vi "Multiple Sessions with a Raspberry Pi.vi"() -> ()   [LabVIEW 2018]
doc: "Creates multiple, parallel sessions with a Raspberry Pi."
uses:
  Toolkit/Channel/Channel.lvclass/Channel.ctl
  Toolkit/Session/Session.lvclass/Session.ctl
  Toolkit/SSH/SSH.lvclass/SSH.ctl
  Toolkit/Session/Utility/Read Shared Library.vi
  Toolkit/SSH/Utility/Read Shared Library.vi
  Toolkit/Session/Support/Create from SSH.vi
  Toolkit/Session/Support/Password Authentication.vi
  Toolkit/Channel/Support/Create from Session.vi
  Toolkit/Support/Check Status.vi
  Toolkit/Channel/Support/Destroy to Session.vi
  Toolkit/Session/Support/Destroy to SSH.vi
  Toolkit/SSH/SSH.lvclass
  Toolkit/Session/Session.lvclass
  Toolkit/Channel/Channel.lvclass
panel:
  out "Login Message Size 2":i32 caption="Login Size"
  out "Login Message 2":string
  out "Login Message Size 1":i32 caption="Login Size"
  in  "Max Login Message Size":u64=1024 caption="Max Login Size"
  out "Response 2 Size":i32 caption="Response Size"
  in  "Command 2 Max Response Size":u64=1024 caption="Max Response Size"
  out "Response 1 Size":i32 caption="Response Size"
  in  "Command 1 Max Response Size":u64=1024 caption="Max Response Size"
  in  "Timeout":i32=1000 caption="Timeout (ms)"
  out "Login Message 1":string
  out "Response 2":string
  in  "Command 2":string="echo \"Hello World from the second command!\""
  out "Response 1":string
  in  "Command 1":string="echo \"Hello World from the first command!\""
  in  "Raspberry Pi Address":string="raspberrypi.local"
  in  "Password":string
  in  "Username":string="pi"
  # "Overview: Demonstrates creating multiple, parallel sessions with a Raspberry Pi\nInstructions:\n1. Change the Raspberry Pi Address from the mDNS default to another mDNS or the IP address of the Raspberry Pi if needed.\n2. Change the username from the default Raspberry Pi user if needed.\n3. Enter the password for the Raspberry Pi user.\n4. Run this VI.\n5. Observe the login message from the Raspberry Pi.\n6. Observe \"Hello World from the first command!\" and \"Hello World from the second command!\" for Response 1 and 2, respectively.\n7. Change Command 1 and Command 2.\n8. Rerun this VI.\n9. Observe the responses for Command 1 and Command 2, respectively."
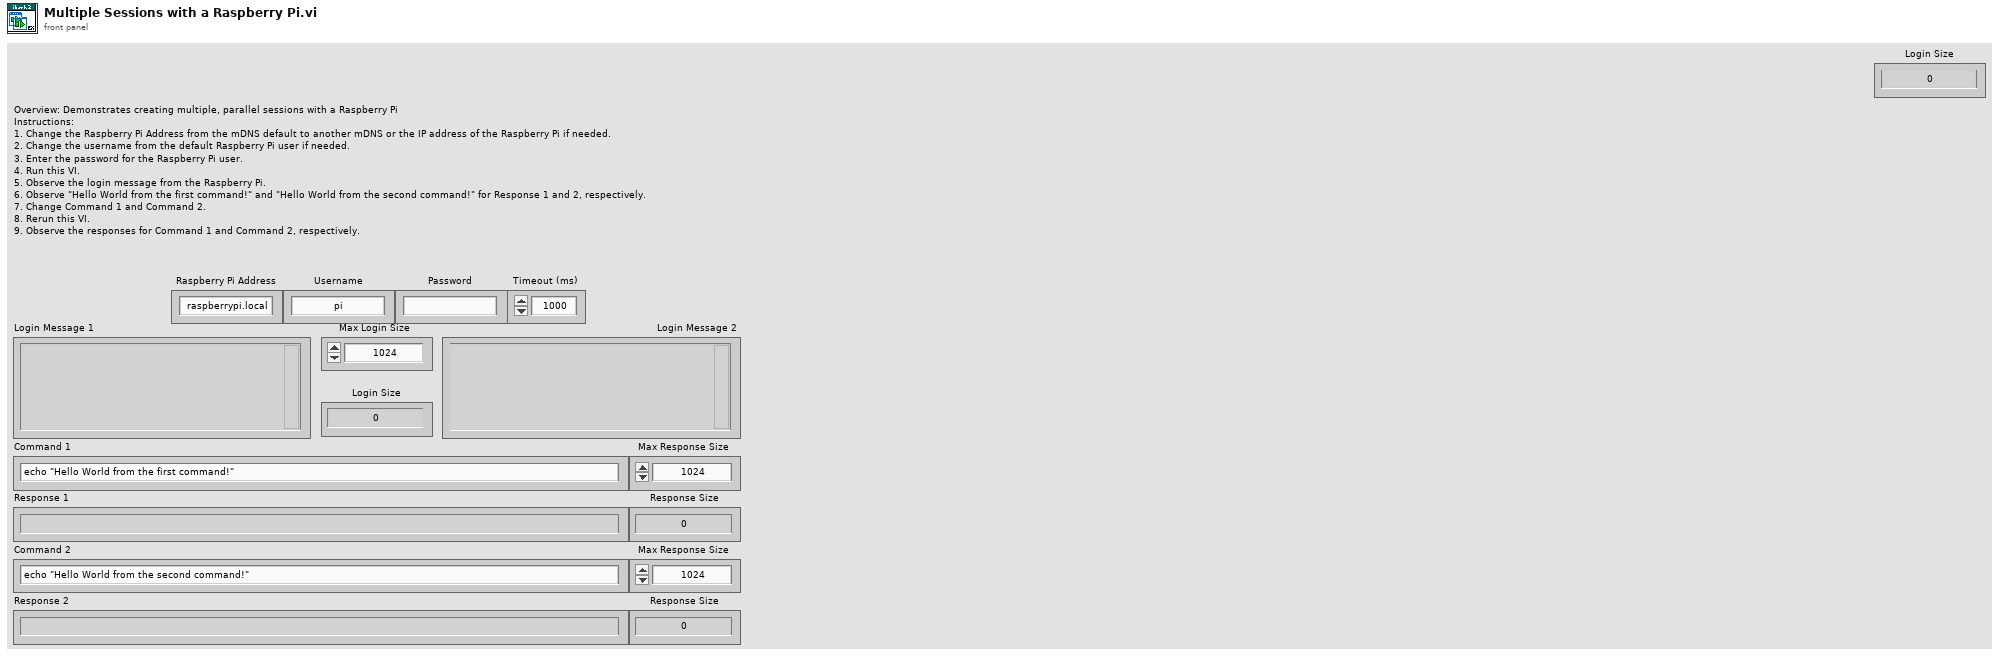
[diagram p1: front panel]
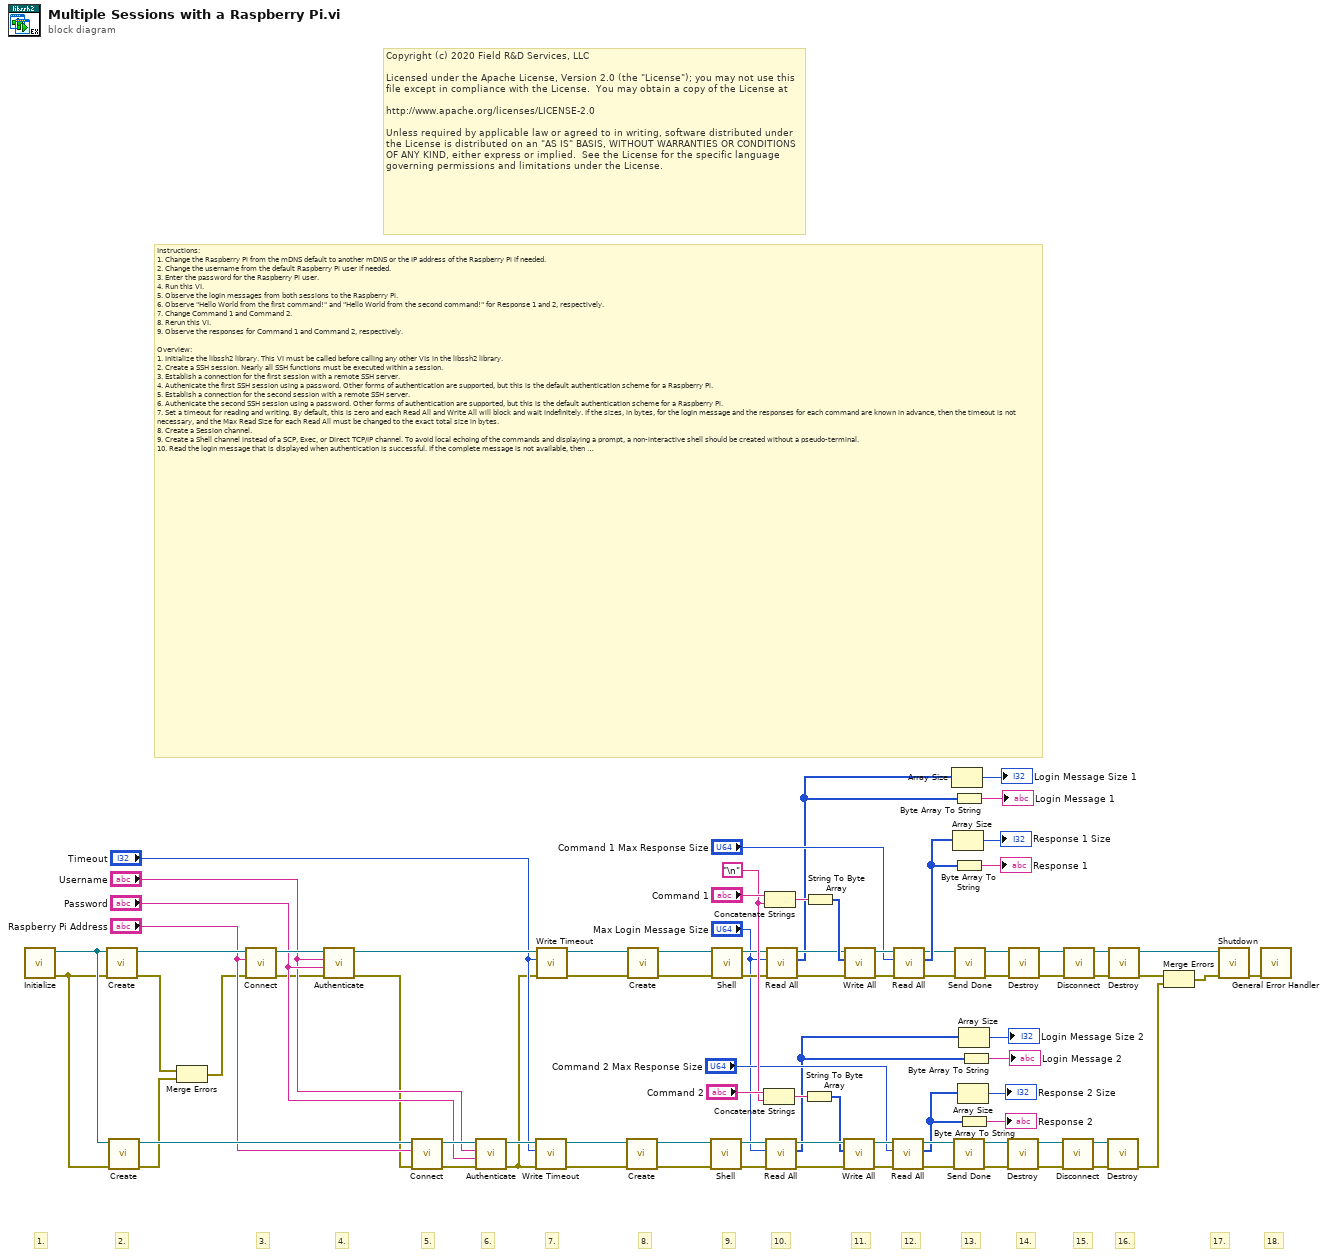
[diagram p0: block diagram]
diagram:
  w62 = "\n"
  # "18."
  # "17."
  # "16."
  # "Copyright (c) 2020 Field R&D Services, LLC\n\nLicensed under the Apache License, Version 2.0 (the \"License\"); you may not use this file except in compliance with the License.  You may obtain a copy of the License at\n\nhttp://www.apache.org/licenses/LICENSE-2.0\n\nUnless required by applicable law or agreed to in writing, software distributed under the License is distributed on an \"AS IS\" BASIS, WITHOUT WARRANTIES OR CONDITIONS OF ANY KIND, either express or implied.  See the License for the specific language governing permissions and limitations under the License."
  # "15."
  # "14."
  # "13."
  # "12."
  # "11."
  # "10."
  # "9."
  # "8."
  # "7."
  # "6."
  # "5."
  # "4."
  # "3."
  # "2."
  # "1."
  # "Instructions:\n1. Change the Raspberry Pi from the mDNS default to another mDNS or the IP address of the Raspberry Pi if needed.\n2. Change the username from the default Raspberry Pi user if needed.\n3. Enter the password for the Raspberry Pi user.\n4. Run this VI.\n5. Observe the login messages from both sessions to the Raspberry Pi.\n6. Observe \"Hello World from the first command!\" and \"Hello World from the second command!\" for Response 1 and 2, respectively.\n7. Change Command 1 and Command 2.\n8. Rerun this VI.\n9. Observe the responses for Command 1 and Command 2, respectively.\n\nOverview:\n1. Initialize the libssh2 library. This VI must be called before calling any other VIs in the libssh2 library.\n2. Create a SSH session. Nearly all SSH functions must be executed within a session.\n3. Establish a connection for the first session with a remote SSH server.\n4. Authenicate the first SSH session using a password. Other forms of authentication are supported, but this is the default authentication scheme for a Raspberry Pi. \n5. Establish a connection for the second session with a remote SSH server.\n6. Authenicate the second SSH session using a password. Other forms of authentication are supported, but this is the default authentication scheme for a Raspberry Pi. \n7. Set a timeout for reading and writing. By default, this is zero and each Read All and Write All will block and wait indefinitely. If the sizes, in bytes, for the login message and the responses for each command are known in advance, then the timeout is not necessary, and the Max Read Size for each Read All must be changed to the exact total size in bytes. \n8. Create a Session channel. \n9. Create a Shell channel instead of a SCP, Exec, or Direct TCP/IP channel. To avoid local echoing of the commands and displaying a prompt, a non-interactive shell should be created without a pseudo-terminal.\n10. Read the login message that is displayed when authentication is successful. If the complete message is not available, then the Timeout will need to be modified.\n11. Execute command 1 by writing it to the Shell channel. The Command 1 Max Response Size is the maximum response size in bytes (B) from the output of executing Command 1. If Timeout is zero (0), then this value must be the exact number of bytes to avoid stalling and waiting indefinitely.\n12. Read the first response. If Timeout is zero (0), then this value will match the Command 1 Max Response Size value.\n13. Signal completion of the Session channel to the remote server. Not strictly required, but it is good practice. \n14. Destroy the Session channel. Since the \"Create\" VI is used, the complementary \"Destroy\" VI must be used to free resources within the libssh2 library.  \n15. Disconnect from the remote SSH server. \n16. Destroy the session to free resources within the libssh2 library.\n17. Shutdown the libssh2 library. This VI must be last VI called for the libssh2 library. No other libssh2 VIs should be called once this VI is executed.\n18. Provide some error handling and reporting. Libssh2 errors will be in the -8100 range while warnings will be in the 5000 range."
  n1 = call "Initialize.vi"() -> ("Error Out"=w6:errorcluster, "SSH"=w45:refnum<class "SSH.lvclass">)  [unwired: 10 in]
  n2 = call-poly "Create.vi"("Error In"=w6, "SSH"=w45) -> ("Error Out"=w5:errorcluster, "Sesssion"=w82:refnum<class "Session.lvclass">)  [unwired: 8 in]
  n3 = call-poly "Create.vi"("Error In"=w6, "SSH"=w45) -> ("Error Out"=w4:errorcluster, "Sesssion"=w42:refnum<class "Session.lvclass">)  [unwired: 8 in]
  n4 = Merge Errors(w5, w4) -> (w3:errorcluster)
  n5 = call "Connect.vi"("Error In"=w3, "Address"="Raspberry Pi Address", "Session In"=w82) -> ("Error Out"=w7:errorcluster, "Sesssion Out"=w81:refnum<class "Session.lvclass">)  [unwired: 7 in]
  n6 = call-poly "Authenticate.vi"("Error In"=w7, "Password"="Password", "Username"="Username", "Session In"=w81) -> ("Error Out"=w2:errorcluster, "Sesssion Out"=w55:refnum<class "Session.lvclass">)  [unwired: 6 in]
  n7 = call "Connect.vi"("Error In"=w2, "Address"="Raspberry Pi Address", "Session In"=w42) -> ("Error Out"=w40:errorcluster, "Sesssion Out"=w41:refnum<class "Session.lvclass">)  [unwired: 7 in]
  n8 = call-poly "Authenticate.vi"("Error In"=w40, "Password"="Password", "Username"="Username", "Session In"=w41) -> ("Error Out"=w1:errorcluster, "Sesssion Out"=w39:refnum<class "Session.lvclass">)  [unwired: 6 in]
  n9 = call "Write Timeout.vi"("Error In"=w1, "Timeout"="Timeout", "Session In"=w39) -> ("Error Out"=w37:errorcluster, "Sesssion Out"=w38:refnum<class "Session.lvclass">)  [unwired: 7 in]
  n10 = call "Write Timeout.vi"("Error In"=w1, "Timeout"="Timeout", "Session In"=w55) -> ("Error Out"=w54:errorcluster, "Sesssion Out"=w53:refnum<class "Session.lvclass">)  [unwired: 7 in]
  n11 = call-poly "Create.vi"("Error In"=w37, "Session"=w38) -> ("Error Out"=w35:errorcluster, "Channel"=w36:refnum<class "Channel.lvclass">)  [unwired: 8 in]
  n12 = call-poly "Create.vi"("Error In"=w54, "Session"=w53) -> ("Error Out"=w60:errorcluster, "Channel"=w61:refnum<class "Channel.lvclass">)  [unwired: 8 in]
  n13 = call "Shell.vi"("Error In"=w35, "Channel In"=w36) -> ("Error Out"=w33:errorcluster, "Channel Out"=w34:refnum<class "Channel.lvclass">)  [unwired: 8 in]
  n14 = call "Shell.vi"("Error In"=w60, "Channel In"=w61) -> ("Error Out"=w58:errorcluster, "Channel Out"=w59:refnum<class "Channel.lvclass">)  [unwired: 8 in]
  n15 = Concatenate Strings("Command 2", w62) -> (w63:string)
  n16 = Concatenate Strings("Command 1", w62) -> (w65:string)
  n17 = call "Read All.vi"("Error In"=w33, "Max Read Size"="Max Login Message Size", "Channel In"=w34) -> ("Error Out"=w31:errorcluster, "Data"=w8:u8[], "Channel Out"=w32:refnum<class "Channel.lvclass">)  [unwired: 5 in, 1 out]
  n18 = call "Read All.vi"("Error In"=w58, "Max Read Size"="Max Login Message Size", "Channel In"=w59) -> ("Error Out"=w52:errorcluster, "Data"=w47:u8[], "Channel Out"=w67:refnum<class "Channel.lvclass">)  [unwired: 5 in, 1 out]
  n19 = String To Byte Array(string=w63) -> (unsigned byte array=w17:u8[])
  n20 = String To Byte Array(string=w65) -> (unsigned byte array=w69:u8[])
  n21 = call "Write All.vi"("Error In"=w31, "Data"=w17, "Channel In"=w32) -> ("Error Out"=w29:errorcluster, "Channel Out"=w30:refnum<class "Channel.lvclass">)  [unwired: 5 in, 2 out]
  n22 = call "Write All.vi"("Error In"=w52, "Data"=w69, "Channel In"=w67) -> ("Error Out"=w57:errorcluster, "Channel Out"=w68:refnum<class "Channel.lvclass">)  [unwired: 5 in, 2 out]
  n23 = call "Read All.vi"("Error In"=w29, "Max Read Size"="Command 2 Max Response Size", "Channel In"=w30) -> ("Error Out"=w27:errorcluster, "Data"=w18:u8[], "Channel Out"=w28:refnum<class "Channel.lvclass">)  [unwired: 5 in, 1 out]
  n24 = call "Read All.vi"("Error In"=w57, "Max Read Size"="Command 1 Max Response Size", "Channel In"=w68) -> ("Error Out"=w43:errorcluster, "Data"=w51:u8[], "Channel Out"=w44:refnum<class "Channel.lvclass">)  [unwired: 5 in, 1 out]
  n25 = Array Size(array=w47) -> (size(s)=→"Login Message Size 1":i32)
  n26 = Array Size(array=w51) -> (size(s)=→"Response 1 Size":i32)
  n27 = Byte Array To String(unsigned byte array=w47) -> (string=→"Login Message 1":string)
  n28 = Byte Array To String(unsigned byte array=w51) -> (string=→"Response 1":string)
  n29 = call "Send Done.vi"("Error In"=w27, "Channel In"=w28) -> ("Error Out"=w25:errorcluster, "Channel Out"=w26:refnum<class "Channel.lvclass">)  [unwired: 8 in]
  n30 = call "Send Done.vi"("Error In"=w43, "Channel In"=w44) -> ("Error Out"=w79:errorcluster, "Channel Out"=w80:refnum<class "Channel.lvclass">)  [unwired: 8 in]
  n31 = Array Size(array=w18) -> (size(s)=→"Response 2 Size":i32)
  n32 = Array Size(array=w8) -> (size(s)=→"Login Message Size 2":i32)
  n33 = Byte Array To String(unsigned byte array=w18) -> (string=→"Response 2":string)
  n34 = Byte Array To String(unsigned byte array=w8) -> (string=→"Login Message 2":string)
  n35 = call-poly "Destroy.vi"("Error In"=w25, "Channel"=w26) -> ("Error Out"=w23:errorcluster, "Session"=w24:refnum<class "Session.lvclass">)  [unwired: 8 in]
  n36 = call-poly "Destroy.vi"("Error In"=w79, "Channel"=w80) -> ("Error Out"=w77:errorcluster, "Session"=w78:refnum<class "Session.lvclass">)  [unwired: 8 in]
  n37 = call "Disconnect.vi"("Error In"=w23, "Session In"=w24) -> ("Error Out"=w21:errorcluster, "Sesssion Out"=w22:refnum<class "Session.lvclass">)  [unwired: 8 in]
  n38 = call "Disconnect.vi"("Error In"=w77, "Session In"=w78) -> ("Error Out"=w75:errorcluster, "Sesssion Out"=w76:refnum<class "Session.lvclass">)  [unwired: 8 in]
  n39 = call-poly "Destroy.vi"("Error In"=w21, "Session"=w22) -> ("Error Out"=w19:errorcluster)  [unwired: 8 in, 1 out]
  n40 = call-poly "Destroy.vi"("Error In"=w75, "Session"=w76) -> ("Error Out"=w73:errorcluster, "SSH"=w74:refnum<class "SSH.lvclass">)  [unwired: 8 in]
  n41 = Merge Errors(w73, w19) -> (w20:errorcluster)
  n42 = call "Shutdown.vi"("Error In"=w20, "SSH"=w74) -> ("Error Out"=w71:errorcluster)  [unwired: 9 in]
  n43 = call <vilib>:"General Error Handler.vi"("error in (no error)"=w71) -> ()  [unwired: 10 in, 5 out]
